vi "ExampleAll.vi"() -> ()   [LabVIEW 2009]
uses:
  Shamrock.llb/shamrock_flipperPort_typedef.ctl
  Shamrock.llb/shamrock_lipperMirror_typedef.ctl
  C/Program Files (x86)/National Instruments/LabVIEW 2018/user.lib/Shamrock.llb/shamrock_autoSlit_typedef.ctl
panel:
  in  "Device":i32 min=0 max=1
  in  "Tab Control":T1(tab)
  in  "Grating Offset":i32
  out "SetGratingOffset":string
  in  "Detector Offset":i32
  out "SetDetectorOffset":string
  out "WavelengthReset":string
  out "SetGrating":string
  in  "Grating":i32
  in  "Turret":i32
  out "SetTurret":string
  in  "SetGratingOffset":bool
  in  "SetDetectorOffset":bool
  in  "WavelengthReset":bool
  in  "SetGrating":bool
  in  "SetTurret":bool
  out "blaze":string
  out "Grating Offset":i32
  out "Detector Offset":i32
  out "offset":i32
  out "home":i32
  out "lines/mm":dbl format="%.2f"
  out "Grating":i32
  out "No Gratings":i32
  out "Turret":i32
  out "Is Grating ?":string
  out "GetGratingOffset":string
  out "GetDetectorOffset":string
  out "GetGratingInfo":string
  out "GetGrating":string
  out "GetNumberGratings":string
  out "GetTurret":string
  out "GratingIsPresent":string
  out "GetCalibration":string
  out "SetNumberPixels":string
  out "SetPixelWidth":string
  out "Max Dispersion":sgl
  out "Min Dispersion":sgl
  in  "Number Pixels":u32 caption="Numeric"
  in  "Pixel Width":sgl caption="Numeric" format="%_3g"
  out "GotoZeroOrder":string
  out "SetWavelength":string
  in  "Wavelength":dbl format="%.2f"
  in  "GoToZeroOrder":bool
  out "Max Wavelength":dbl format="%.2f"
  out "Min Wavelength":dbl format="%.2f"
  out "Is Wavelength ?":string
  out "WavelengthIsPresent":string
  out "GetWavelengthLimits":string
  out "At Zero Order ?":string
  out "AtZeroOrder":string
  out "Wavelength":dbl format="%.2f"
  in  "SetWavelength 2":bool
  out "GetWavelength":string
  out "SetSlitZeroPosition":string
  out "GetSlitZeroPosition":string
  in  "SlitZeroPositionSet":bool caption="SetSlitZeroPosition"
  in  "SlitZeroPositionGet":bool
  in  "SlitZeroPosition":i32
  in  "Reset Slit":bool
  out "ResetSlit":string
  out "Getslit":string
  in  "Slit Width":dbl format="%.2f"
  in  "SetSlit":bool
  out "Slit width(mm)":dbl format="%.2f"
  out "GetSlit":string
  out "SlitIsPresent retun code":string
  in  "Slit":T2
  out "Is Slit Present?":bool
  in  "Mode":i32
  in  "SetShutter":bool
  out "Is Mode Possible ?":string
  out "Shutter":i32
  out "Is Shutter ?":string
  out "SetShutter":string
  out "IsModePossible":string
  out "GetShutter":string
  out "ShutterIsPresent":string
  in  "Flipper Port":T3
  out "High":dbl format="%.2f"
  in  "FlipperReset":bool
  out "FlipperReset":string
  in  "SetPort":bool
  out "Low":dbl format="%.2f"
  out "Port":T3
  out "Is Flipper ?":string
  out "SetPort":string
  out "GetCCDLimits":string
  out "GetPort":string
  out "FlipperIsPresent":string
  out "GetFlipperMirror":string
  in  "FlipperSelect":bool
  in  "Flipper Mirror":T4
  in  "Filter info":string caption="String"
  out "Filter Info":string
  in  "SetFilterInfo":bool
  out "SetFilterInfo":string
  in  "Filter":i32
  in  "SetFilter":bool
  out "Filter":i32
  out "Is Filter ?":string
  out "SetFilter":string
  out "GetFilterInfo":string
  out "GetFilter":string
  out "FilterIsPresent":string
  in  "Reset Focus Mirror":bool
  out "Is Focus Mirror Present?":bool
  out "Focus Mirror Max Steps":i32
  in  "Focus Mirror -":bool
  in  "Focus":i32
  in  "Focus Mirror +":bool
  out "Focus Mirror Position":i32
  out "GetFocusMirrorMaxSteps":string
  out "GetFocusMirror":string
  out "FocusMirrorIsPresent":string
  in  "Line":i32
  out "Line 2":i32
  in  "State":i32
  in  "Set Accessory":bool
  out "Line 1":i32
  out "Is Accessory ?":string
  out "SetAccessory":string
  out "GetAccessory":string
  out "AccessoryIsPresent":string
  in  "Set Params":bool
  out "Set Optical Parameters":string
  in  "Focal tilt":dbl format="%.2f"
  in  "Angular deviation":dbl format="%.2f"
  in  "Focal length":dbl format="%.4f"
  out "Initializing":bool
  in  "STOP if TRUE":bool
  out "Focal tilt":dbl format="%.2f"
  out "Angular deviation":dbl format="%.2f"
  out "Focal length":dbl format="%.4f"
  out "Serial Number":string
  out "No of devices":i32
  out "GetOpticalParameters":string
  out "GetSerialNumber":string
  out "GetNumberDevices":string
  out "Close":string
  out "Initialize":string
  # "INITIALIZATION"
  # "SDK RETURN VALUES"
  # "SHAMROCK PARAMETERS"
  # "ACTIONS"
  # "SDK RETURN VALUES"
  # "SHAMROCK PARAMETERS"
  # "ACTIONS"
  # "SDK RETURN VALUES"
  # "SHAMROCK PARAMETERS"
  # "ACTIONS"
  # "nm"
  # "Dispersion range"
  # "SDK RETURN VALUES"
  # "SHAMROCK PARAMETERS"
  # "ACTIONS"
  # "mm"
  # "SetZero position"
  # "SDK RETURN VALUES"
  # "SHAMROCK PARAMETERS"
  # "ACTIONS"
  # "( 0:Closed / 1:Open )"
  # "SDK RETURN VALUES"
  # "SHAMROCK PARAMETERS"
  # "ACTIONS"
  # "SDK RETURN VALUES"
  # "SHAMROCK PARAMETERS"
  # "ACTIONS"
  # "SDK RETURN VALUES"
  # "SHAMROCK PARAMETERS"
  # "ACTIONS"
  # "SDK RETURN VALUES"
  # "SHAMROCK PARAMETERS"
  # "ACTIONS"
  # "line"
  # "to state"
  # "SDK RETURN VALUES"
  # "SHAMROCK PARAMETERS"
  # "ACTIONS"
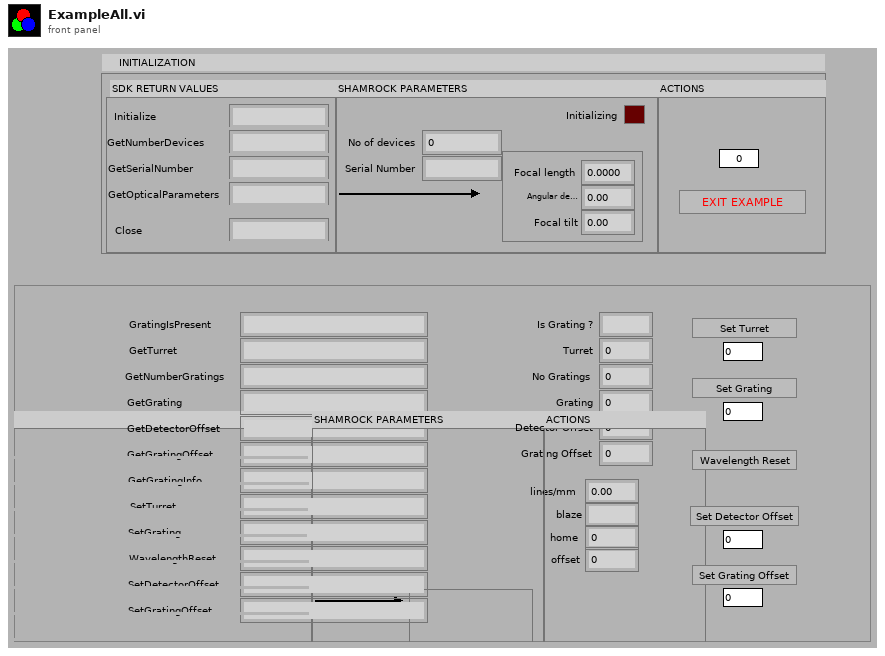
[diagram p1: front panel]
types:
  T1 = enum32{"GRATINGS", "WAVELENGTH", "INPUT & OUTPUT SLIT", "SHUTTER", "FLIPPER", "FILTER", "FOCUS", "ACCESSORY", "OPTICALPARAMS"}
  T2 = typedef "shamrock_autoSlit_typedef.ctl" = enum32{"Reserved (0)", "INPUT SIDE", "INPUT DIRECT", "OUTPUT SIDE", "OUTPUT DIRECT"}
  T3 = typedef "shamrock_flipperPort_typedef.ctl" = enum32{"DIRECT PORT", "SIDE PORT"}
  T4 = typedef "shamrock_lipperMirror_typedef.ctl" = enum32{"Reserved (0)", "INPUT MIRROR", "OUTPUT MIRROR"}
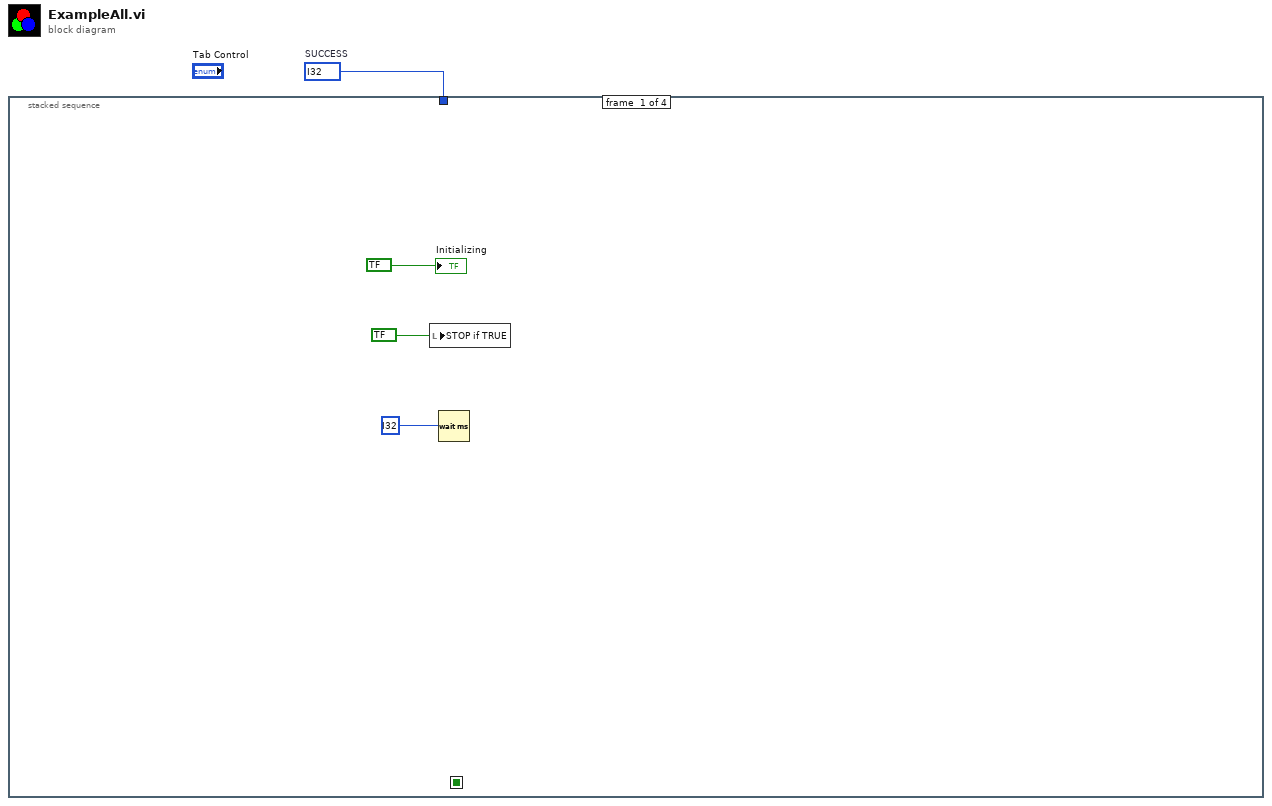
[diagram p0: block diagram]
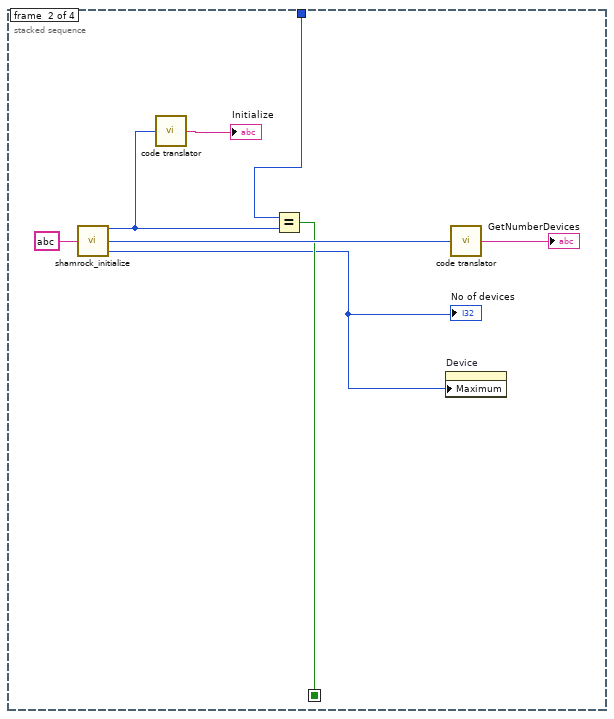
[diagram p2: hidden frame]
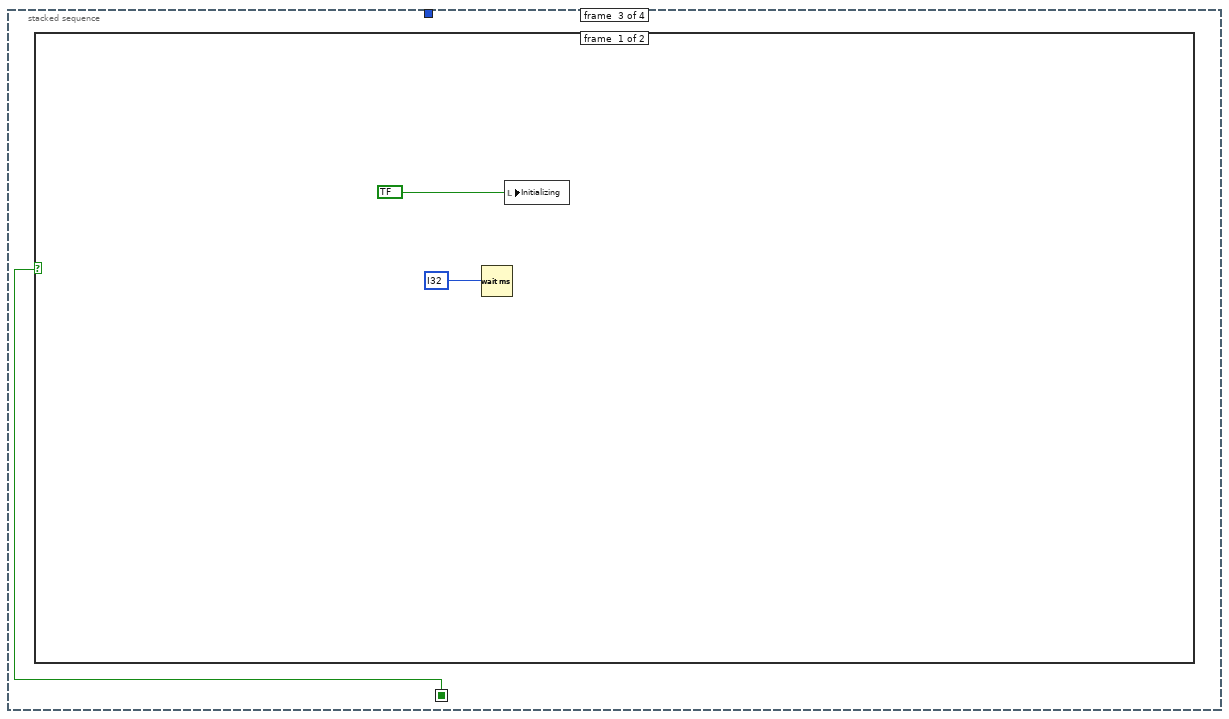
[diagram p3: hidden frame]
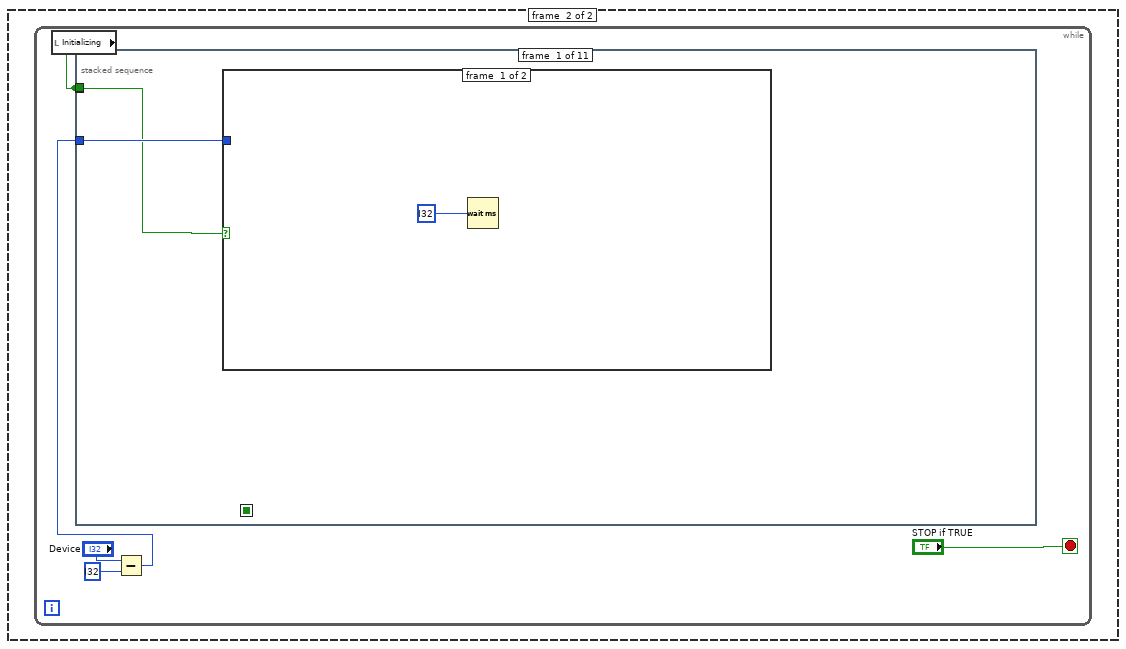
[diagram p4: hidden frame]
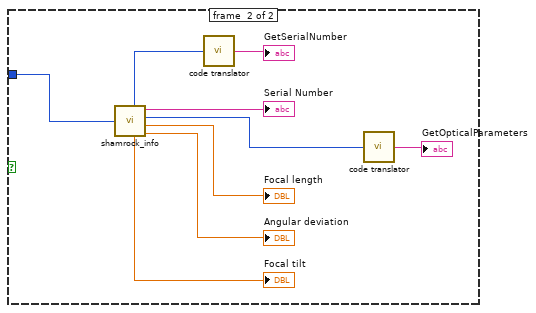
[diagram p5: hidden frame]
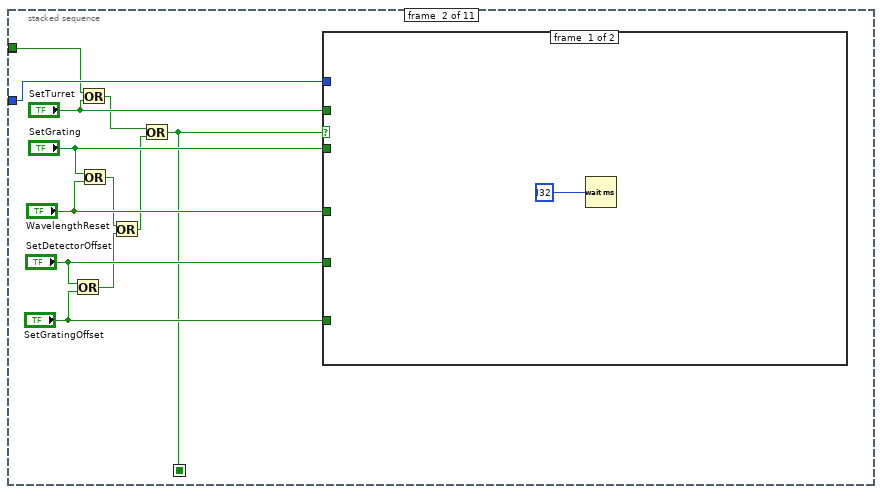
[diagram p6: hidden frame]
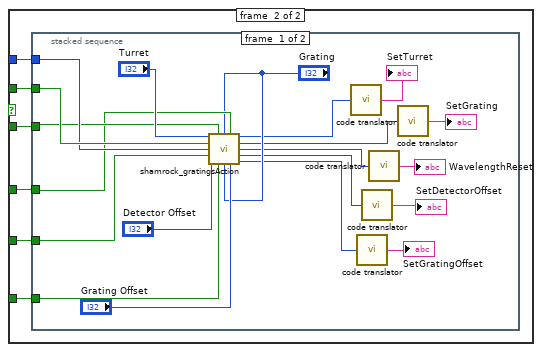
[diagram p7: hidden frame]
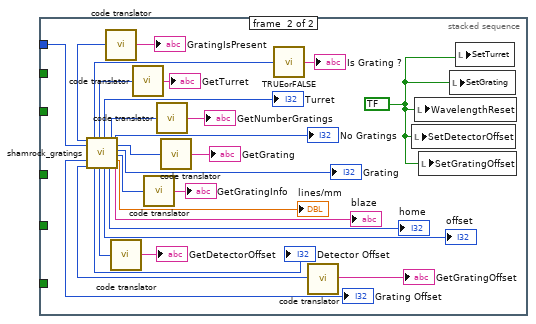
[diagram p8: hidden frame]
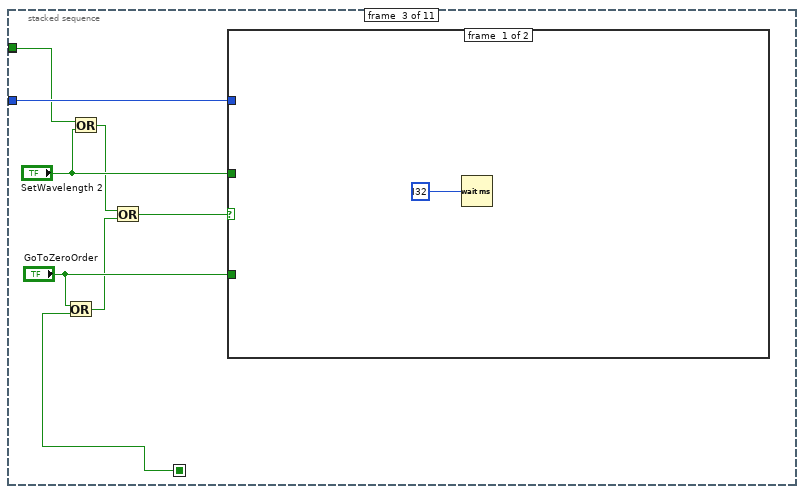
[diagram p9: hidden frame]
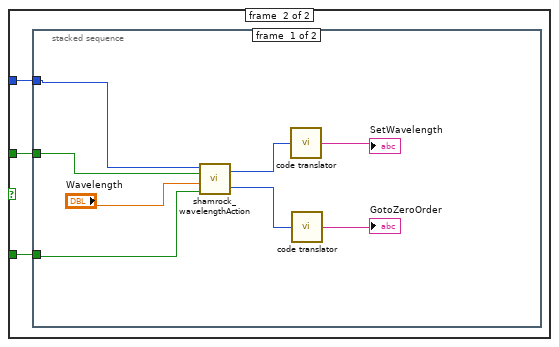
[diagram p10: hidden frame]
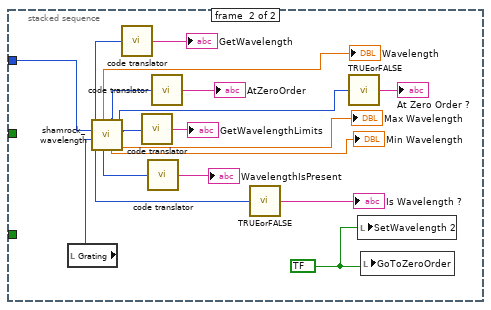
[diagram p11: hidden frame]
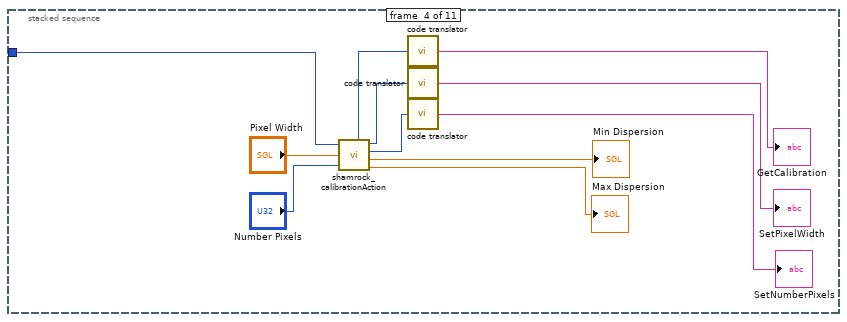
[diagram p12: hidden frame]
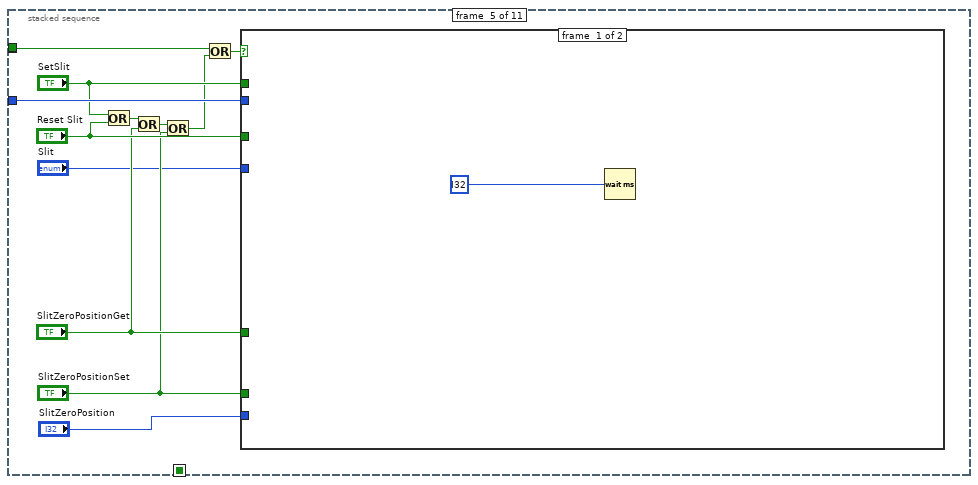
[diagram p13: hidden frame]
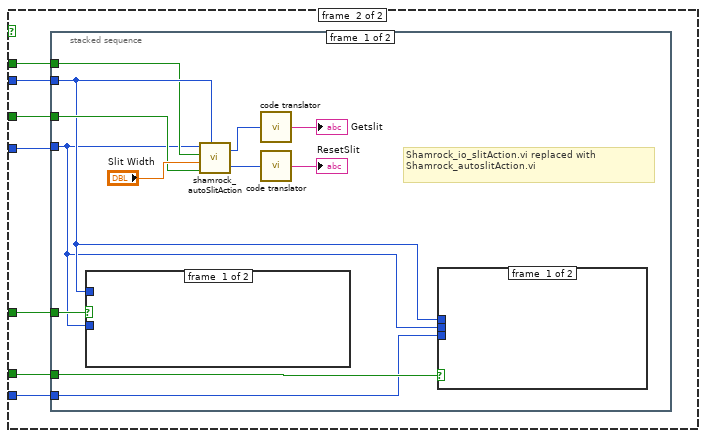
[diagram p14: hidden frame]
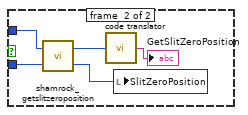
[diagram p15: hidden frame]
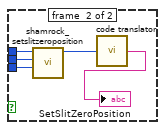
[diagram p16: hidden frame]
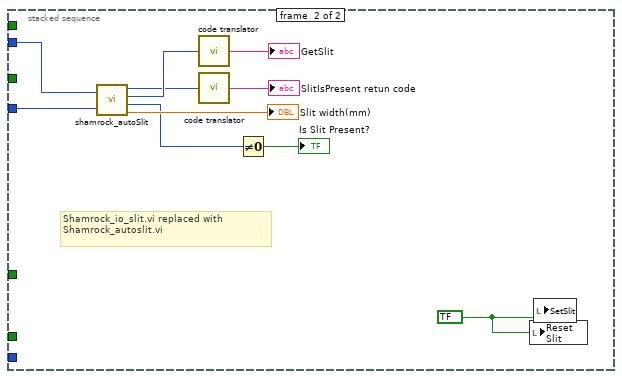
[diagram p17: hidden frame]
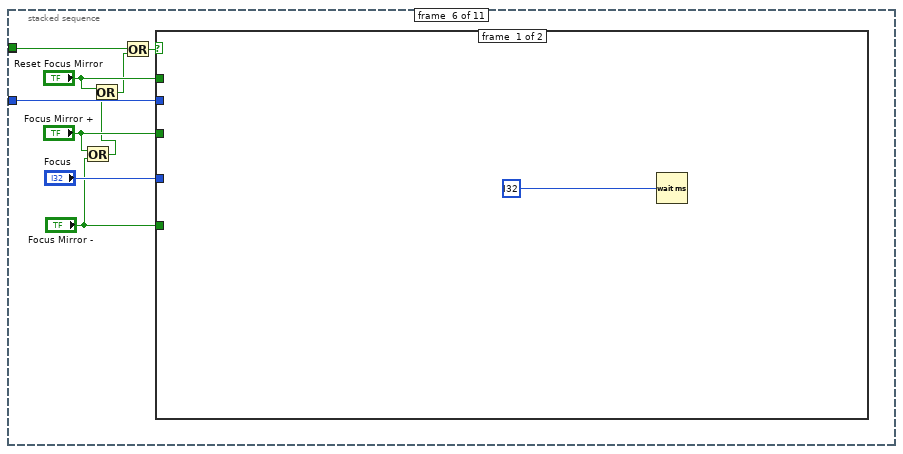
[diagram p18: hidden frame]
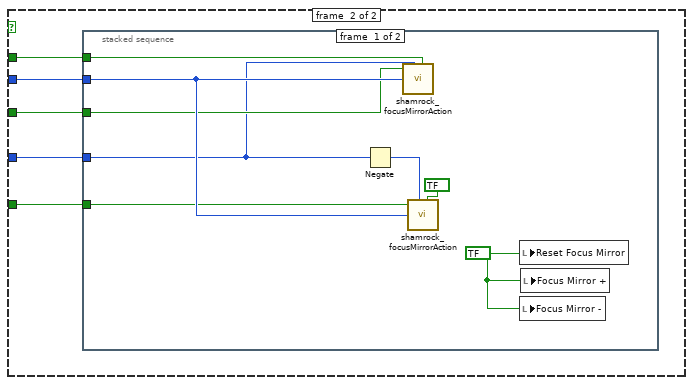
[diagram p19: hidden frame]
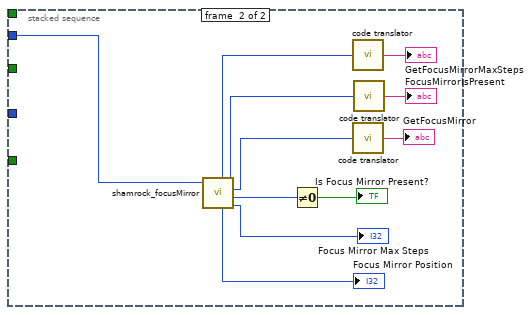
[diagram p20: hidden frame]
diagram:
  w1 = i32 ?  # SUCCESS
  n1 = stacked-sequence {
    seq-local: [_ w6 _ _] -> [_ _ w13 _]
    tunnel: w1 -> [_ w12 _ _]
    frame #0 {
      n2 = local write "STOP if TRUE"(bool ?) -> ()
      n3 = Wait (ms)(milliseconds to wait=i32 ?) -> ()  [unwired: 1 out]
      "Initializing" <- bool ?
    }
    frame #1 {
      n4 = call "shamrock_initialize.vi"("Initialization path"=string ?) -> ("Initialize"=w9:u32, "GetNumberDevices"=w8:u32, "No of devices"=w5:i32)
      "No of devices" <- w5
      n5 = call "code translator.vi"("Error code"=w9) -> ("Error description"=→"Initialize":string)
      n6 = Equal?(x=w12, y=w9) -> (x = y?=w6:bool)
      n7 = property on="Device" class="DigNum (strict)"("Maximum"=w5) -> ()  [unwired: 2 in, 2 out]
      n8 = call "code translator.vi"("Error code"=w8) -> ("Error description"=→"GetNumberDevices":string)
    }
    frame #2 {
      n9 = case shown="True" w13 {
        frame #0 {
          n10 = Wait (ms)(milliseconds to wait=i32 ?) -> ()  [unwired: 1 out]
          n11 = local write "Initializing"(bool ?) -> ()
        }
        frame #1 {
          n12 = while {
            stop <- "STOP if TRUE" stop-if-true
            n13 = local read "Initializing"() -> (w16:bool)
            n14 = Subtract(x="Device", y=i32 ?) -> (x-y=w19:i32)
            n15 = stacked-sequence {
              seq-local: [_ w33 _ _ _ _ _ _ _ _ _] -> [_ _ w105 _ _ _ _ _ _ _ _]
              tunnel: w19 -> [w22 w44 w106 w138 w159 w208 w237 w267 w302 w331 w355]
              tunnel: w16 -> [w21 w36 w102 _ w155 w201 w234 _ w297 w328 _]
              tunnel: w16 -> [_ _ _ _ _ _ _ w263 _ _ _]
              frame #0 {
                n16 = case shown="True" w21 {
                  tunnel: w22 -> [_ w24]
                  frame #0 {
                    n17 = Wait (ms)(milliseconds to wait=i32 ?) -> ()  [unwired: 1 out]
                  }
                  frame #1 {
                    n18 = call "shamrock_info.vi"("Device No"=w24) -> ("GetSerialNumber"=w28:u32, "Focal tilt"=→"Focal tilt":sgl, "Serial Number"=→"Serial Number":string, "GetOpticalParameters"=w26:u32, "Focal length"=→"Focal length":sgl, "Angular deviation"=→"Angular deviation":sgl)
                    n19 = call "code translator.vi"("Error code"=w28) -> ("Error description"=→"GetSerialNumber":string)
                    n20 = call "code translator.vi"("Error code"=w26) -> ("Error description"=→"GetOpticalParameters":string)
                  }
                }
              }
              frame #1 {
                n21 = Or(x="SetDetectorOffset", y="SetGratingOffset") -> (x .or. y?=w38:bool)
                n22 = Or(x=w36, y="SetTurret") -> (x .or. y?=w35:bool)
                n23 = Or(x="SetGrating", y="WavelengthReset") -> (x .or. y?=w39:bool)
                n24 = Or(x=w39, y=w38) -> (x .or. y?=w34:bool)
                n25 = Or(x=w35, y=w34) -> (x .or. y?=w33:bool)
                n26 = case shown="True" w33 {
                  tunnel: w44 -> [_ w51]
                  tunnel: "SetDetectorOffset" -> [_ w50]
                  tunnel: "SetGratingOffset" -> [_ w49]
                  tunnel: "SetGrating" -> [_ w48]
                  tunnel: "WavelengthReset" -> [_ w47]
                  tunnel: "SetTurret" -> [_ w46]
                  frame #0 {
                    n27 = Wait (ms)(milliseconds to wait=i32 ?) -> ()  [unwired: 1 out]
                  }
                  frame #1 {
                    n28 = stacked-sequence {
                      tunnel: w46 -> [w70 _]
                      tunnel: w51 -> [w69 w89]
                      tunnel: w48 -> [w64 _]
                      tunnel: w47 -> [w63 _]
                      tunnel: w50 -> [w68 _]
                      tunnel: w49 -> [w66 _]
                      frame #0 {
                        n29 = call "shamrock_gratingsAction.vi"("WavelengthReset"=w63, "Grating Offset"="Grating Offset", 7:"Grating"="Grating", 8:"Grating"="Grating", "SetGrating"=w64, "SetGratingOffset"=w66, "Turret"="Turret", "SetTurret"=w70, "Device No"=w69, "SetDetectorOffset"=w68, "Detector Offset"="Detector Offset") -> ("SetTurret"=w61:u32, "SetGrating"=w59:u32, "WavelengthReset"=w56:u32, "SetDetectorOffset"=w54:u32, "SetGratingOffset"=w53:u32)
                        n30 = call "code translator.vi"("Error code"=w61) -> ("Error description"=→"SetTurret":string)
                        n31 = call "code translator.vi"("Error code"=w53) -> ("Error description"=→"SetGratingOffset":string)
                        n32 = call "code translator.vi"("Error code"=w54) -> ("Error description"=→"SetDetectorOffset":string)
                        n33 = call "code translator.vi"("Error code"=w56) -> ("Error description"=→"WavelengthReset":string)
                        n34 = call "code translator.vi"("Error code"=w59) -> ("Error description"=→"SetGrating":string)
                      }
                      frame #1 {
                        w98 = bool ?
                        n35 = call "shamrock_gratings.vi"("Device No"=w89) -> ("No Gratings"=→"No Gratings":i32, "GetNumberGratings"=w83:u32, "Turret"=→"Turret":i32, "GetTurret"=w85:u32, "0:FALSE / 1:TRUE"=w73:i32, "GratingIsPresent"=w87:u32, "GetGrating"=w81:u32, "Grating"=→"Grating":i32, "GetGratingInfo"=w79:u32, "lines/mm"=→"lines/mm":dbl, "Grating Offset"=→"Grating Offset":i32, "blaze"=→"blaze":string, "home"=→"home":i32, "offset"=→"offset":i32, "GetDetectorOffset"=w77:u32, "Detector Offset"=→"Detector Offset":i32, "GetGratingOffset"=w75:u32)  [unwired: 1 in, 1 out]
                        n36 = call "code translator.vi"("Error code"=w87) -> ("Error description"=→"GratingIsPresent":string)
                        n37 = call "code translator.vi"("Error code"=w77) -> ("Error description"=→"GetDetectorOffset":string)
                        n38 = call "code translator.vi"("Error code"=w85) -> ("Error description"=→"GetTurret":string)
                        n39 = call "code translator.vi"("Error code"=w79) -> ("Error description"=→"GetGratingInfo":string)
                        n40 = call "code translator.vi"("Error code"=w83) -> ("Error description"=→"GetNumberGratings":string)
                        n41 = call "code translator.vi"("Error code"=w81) -> ("Error description"=→"GetGrating":string)
                        n42 = call "TRUEorFALSE.vi"("bool number"=w73) -> ("String"=→"Is Grating ?":string)
                        n43 = call "code translator.vi"("Error code"=w75) -> ("Error description"=→"GetGratingOffset":string)
                        n44 = local write "SetDetectorOffset"(w98) -> ()
                        n45 = local write "WavelengthReset"(w98) -> ()
                        n46 = local write "SetGratingOffset"(w98) -> ()
                        n47 = local write "SetGrating"(w98) -> ()
                        n48 = local write "SetTurret"(w98) -> ()
                      }
                    }
                  }
                }
              }
              frame #2 {
                n49 = Or(x="GoToZeroOrder", y=w105) -> (x .or. y?=w100:bool)
                n50 = Or(x=w102, y="SetWavelength 2") -> (x .or. y?=w101:bool)
                n51 = Or(x=w101, y=w100) -> (x .or. y?=w99:bool)
                n52 = case shown="True" w99 {
                  tunnel: "SetWavelength 2" -> [_ w110]
                  tunnel: "GoToZeroOrder" -> [_ w109]
                  tunnel: w106 -> [_ w108]
                  frame #0 {
                    n53 = Wait (ms)(milliseconds to wait=i32 ?) -> ()  [unwired: 1 out]
                  }
                  frame #1 {
                    n54 = stacked-sequence {
                      tunnel: w110 -> [w116 _]
                      tunnel: w109 -> [w117 _]
                      tunnel: w108 -> [w115 w131]
                      frame #0 {
                        n55 = call "shamrock_wavelengthAction.vi"("GoToZeroOrder"=w117, "Wavelength"="Wavelength", "SetWavelength"=w116, "Device No"=w115) -> ("GotoZeroOrder"=w112:u32, "SetWavelength"=w114:u32)
                        n56 = call "code translator.vi"("Error code"=w114) -> ("Error description"=→"SetWavelength":string)
                        n57 = call "code translator.vi"("Error code"=w112) -> ("Error description"=→"GotoZeroOrder":string)
                      }
                      frame #1 {
                        w136 = bool ?
                        n58 = local read "Grating"() -> (w132:i32)
                        n59 = call "shamrock_wavelength.vi"("Grating No"=w132, "Device No"=w131) -> (0:"0:FALSE / 1:TRUE"=w120:i32, "WavelengthIsPresent"=w124:u32, "Min wl"=→"Min Wavelength":dbl, "Max wl"=→"Max Wavelength":dbl, "GetWavelengthLimits"=w126:u32, "GetWavelength"=w130:u32, "Wavelength"=→"Wavelength":dbl, "AtZeroOrder"=w128:u32, 10:"0:FALSE / 1:TRUE"=w122:i32)
                        n60 = call "code translator.vi"("Error code"=w130) -> ("Error description"=→"GetWavelength":string)
                        n61 = call "code translator.vi"("Error code"=w126) -> ("Error description"=→"GetWavelengthLimits":string)
                        n62 = call "code translator.vi"("Error code"=w124) -> ("Error description"=→"WavelengthIsPresent":string)
                        n63 = call "code translator.vi"("Error code"=w128) -> ("Error description"=→"AtZeroOrder":string)
                        n64 = call "TRUEorFALSE.vi"("bool number"=w120) -> ("String"=→"Is Wavelength ?":string)
                        n65 = call "TRUEorFALSE.vi"("bool number"=w122) -> ("String"=→"At Zero Order ?":string)
                        n66 = local write "SetWavelength 2"(w136) -> ()
                        n67 = local write "GoToZeroOrder"(w136) -> ()
                      }
                    }
                  }
                }
              }
              frame #3 {
                n68 = call "shamrock_calibrationAction.vi"("Set Number Pixels"="Number Pixels", "Set Pixel Width"="Pixel Width", "Device No"=w138) -> ("Wavelength Last Pixel"=→"Max Dispersion":sgl, "Wavelength First Pixel"=→"Min Dispersion":sgl, "Set Number Pixels"=w143:u32, "GetCalibration"=w147:u32, "Set Pixel Width"=w145:u32)  [unwired: 1 out]
                n69 = call "code translator.vi"("Error code"=w147) -> ("Error description"=→"GetCalibration":string)
                n70 = call "code translator.vi"("Error code"=w145) -> ("Error description"=→"SetPixelWidth":string)
                n71 = call "code translator.vi"("Error code"=w143) -> ("Error description"=→"SetNumberPixels":string)
              }
              frame #4 {
                n72 = Or(x="SetSlit", y="Reset Slit") -> (x .or. y?=w148:bool)
                n73 = Or(x=w148, y="SlitZeroPositionGet") -> (x .or. y?=w150:bool)
                n74 = Or(x=w150, y="SlitZeroPositionSet") -> (x .or. y?=w151:bool)
                n75 = Or(x=w155, y=w151) -> (x .or. y?=w156:bool)
                n76 = case shown="True" w156 {
                  tunnel: w159 -> [_ w167]
                  tunnel: "SetSlit" -> [_ w166]
                  tunnel: "Reset Slit" -> [_ w165]
                  tunnel: "SlitZeroPositionGet" -> [_ w164]
                  tunnel: "SlitZeroPositionSet" -> [_ w163]
                  tunnel: "SlitZeroPosition" -> [_ w162]
                  tunnel: "Slit" -> [_ w161]
                  frame #0 {
                    n77 = Wait (ms)(milliseconds to wait=i32 ?) -> ()  [unwired: 1 out]
                  }
                  frame #1 {
                    n78 = stacked-sequence {
                      tunnel: w166 -> [w169 _]
                      tunnel: w167 -> [w172 w196]
                      tunnel: w165 -> [w173 _]
                      tunnel: w164 -> [w177 _]
                      tunnel: w163 -> [w176 _]
                      tunnel: w162 -> [w175 _]
                      tunnel: w161 -> [w168 w195]
                      frame #0 {
                        # "Shamrock_io_slitAction.vi replaced with \nShamrock_autoslitAction.vi"
                        n79 = case shown="True" w177 {
                          tunnel: w172 -> [_ w183]
                          tunnel: w168 -> [_ w182]
                          frame #0 {
                          }
                          frame #1 {
                            n80 = call "shamrock_getslitzeroposition.vi"("Slit Index"=w182, "Device No"=w183) -> ("Offset"=w180:i32, "GetSlitZeroPosition"=w181:u32)
                            n81 = call "code translator.vi"("Error code"=w181) -> ("Error description"=→"GetSlitZeroPosition":string)
                            n82 = local write "SlitZeroPosition"(w180) -> ()
                          }
                        }
                        n83 = call "shamrock_autoSlitAction.vi"("Slit"=w168, "SetSlit"=w169, "Slit Width"="Slit Width", "Reset Slit"=w173, "Device No"=w172) -> ("RC_ResetSlit"=w170:u32, "RC_SetSlit"=w171:u32)
                        n84 = call "code translator.vi"("Error code"=w170) -> ("Error description"=→"Getslit":string)
                        n85 = call "code translator.vi"("Error code"=w171) -> ("Error description"=→"ResetSlit":string)
                        n86 = case shown="True" w176 {
                          tunnel: w172 -> [_ w188]
                          tunnel: w168 -> [_ w187]
                          tunnel: w175 -> [_ w186]
                          frame #0 {
                          }
                          frame #1 {
                            n87 = call "shamrock_setslitzeroposition.vi"("Offset"=w186, "Slit Index"=w187, "Device No"=w188) -> ("SetSlitZeroPosition"=w185:u32)  [unwired: 7 in]
                            n88 = call "code translator.vi"("Error code"=w185) -> ("Error description"=→"SetSlitZeroPosition":string)
                          }
                        }
                      }
                      frame #1 {
                        w199 = bool ?
                        # "Shamrock_io_slit.vi replaced with \nShamrock_autoslit.vi"
                        n89 = call "shamrock_autoSlit.vi"("Device No"=w196, "Slit"=w195) -> ("RC_SlitIsPresent"=w192:u32, "RC_GetSlit"=w194:u32, "IsPresent"=w191:i32, "Slit width (mm)"=→"Slit width(mm)":dbl)
                        n90 = call "code translator.vi"("Error code"=w194) -> ("Error description"=→"GetSlit":string)
                        n91 = call "code translator.vi"("Error code"=w192) -> ("Error description"=→"SlitIsPresent retun code":string)
                        n92 = Not Equal To 0?(x=w191) -> (x != 0?=→"Is Slit Present?":bool)
                        n93 = local write "Reset Slit"(w199) -> ()
                        n94 = local write "SetSlit"(w199) -> ()
                      }
                    }
                  }
                }
              }
              frame #5 {
                n95 = Or(x="Focus Mirror +", y="Focus Mirror -") -> (x .or. y?=w203:bool)
                n96 = Or(x="Reset Focus Mirror", y=w203) -> (x .or. y?=w200:bool)
                n97 = Or(x=w201, y=w200) -> (x .or. y?=w202:bool)
                n98 = case shown="True" w202 {
                  tunnel: w208 -> [_ w214]
                  tunnel: "Focus Mirror +" -> [_ w213]
                  tunnel: "Focus Mirror -" -> [_ w212]
                  tunnel: "Focus" -> [_ w211]
                  tunnel: "Reset Focus Mirror" -> [_ w210]
                  frame #0 {
                    n99 = Wait (ms)(milliseconds to wait=i32 ?) -> ()  [unwired: 1 out]
                  }
                  frame #1 {
                    n100 = stacked-sequence {
                      tunnel: w214 -> [w219 w223]
                      tunnel: w213 -> [w218 _]
                      tunnel: w212 -> [w217 _]
                      tunnel: w211 -> [w216 _]
                      tunnel: w210 -> [w215 _]
                      frame #0 {
                        w220 = bool ?
                        n101 = Negate(x=w216) -> (-x=w222:i32)
                        n102 = call "shamrock_focusMirrorAction.vi"("Set Focus Mirror"=w218, "Focus"=w216, "Device No"=w219, "Reset Focus Mirror"=w215) -> ()  [unwired: 5 in, 2 out]
                        n103 = call "shamrock_focusMirrorAction.vi"("Set Focus Mirror"=w217, "Focus"=w222, "Device No"=w219, "Reset Focus Mirror"=bool ?) -> ()  [unwired: 5 in, 2 out]
                        n104 = local write "Reset Focus Mirror"(w220) -> ()
                        n105 = local write "Focus Mirror -"(w220) -> ()
                        n106 = local write "Focus Mirror +"(w220) -> ()
                      }
                      frame #1 {
                        n107 = call "shamrock_focusMirror.vi"("Device No"=w223) -> ("Max Step Position"=→"Focus Mirror Max Steps":i32, "Current Step Position"=→"Focus Mirror Position":i32, "IsPresent"=w233:i32, "RC_GetFocusMirror"=w228:u32, "RC_GetFocusMirrorMax"=w227:u32, "RC_FocusMirrorPresent"=w226:u32)  [unwired: 2 in]
                        n108 = Not Equal To 0?(x=w233) -> (x != 0?=→"Is Focus Mirror Present?":bool)
                        n109 = call "code translator.vi"("Error code"=w227) -> ("Error description"=→"GetFocusMirrorMaxSteps":string)
                        n110 = call "code translator.vi"("Error code"=w228) -> ("Error description"=→"GetFocusMirror":string)
                        n111 = call "code translator.vi"("Error code"=w226) -> ("Error description"=→"FocusMirrorIsPresent":string)
                      }
                    }
                  }
                }
              }
              frame #6 {
                n112 = Or(x=w234, y="SetShutter") -> (x .or. y?=w235:bool)
                n113 = case shown="True" w235 {
                  tunnel: w237 -> [_ w240]
                  tunnel: "SetShutter" -> [_ w239]
                  frame #0 {
                    n114 = Wait (ms)(milliseconds to wait=i32 ?) -> ()  [unwired: 1 out]
                  }
                  frame #1 {
                    n115 = stacked-sequence {
                      seq-local: ["Mode" _] -> [_ w256]
                      tunnel: w240 -> [w243 w257]
                      tunnel: w239 -> [w244 _]
                      frame #0 {
                        n116 = call "shamrock_shutterAction.vi"("Mode"="Mode", "SetShutter"=w244, "Device No"=w243) -> ("SetShutter"=w242:u32)
                        n117 = call "code translator.vi"("Error code"=w242) -> ("Error description"=→"SetShutter":string)
                      }
                      frame #1 {
                        n118 = call "shamrock_shutter.vi"("Device No"=w257, "Mode"=w256) -> ("ShutterIsPresent"=w255:u32, 3:"0:FALSE / 1:TRUE"=w247:i32, 4:"0:FALSE / 1:TRUE"=w248:i32, "GetShutter"=w253:u32, "Shutter"=→"Shutter":i32, "IsModePossible"=w251:u32)
                        n119 = call "code translator.vi"("Error code"=w255) -> ("Error description"=→"ShutterIsPresent":string)
                        n120 = call "code translator.vi"("Error code"=w251) -> ("Error description"=→"IsModePossible":string)
                        n121 = call "code translator.vi"("Error code"=w253) -> ("Error description"=→"GetShutter":string)
                        n122 = call "TRUEorFALSE.vi"("bool number"=w247) -> ("String"=→"Is Mode Possible ?":string)
                        n123 = call "TRUEorFALSE.vi"("bool number"=w248) -> ("String"=→"Is Shutter ?":string)
                        n124 = local write "SetShutter"(bool ?) -> ()
                      }
                    }
                  }
                }
              }
              frame #7 {
                n125 = Or(x="SetPort", y="FlipperReset") -> (x .or. y?=w264:bool)
                n126 = Or(x=w263, y=w264) -> (x .or. y?=w262:bool)
                n127 = Or(x=w262, y="FlipperSelect") -> (x .or. y?=w260:bool)
                n128 = case shown="True" w260 {
                  tunnel: "SetPort" -> [_ w272]
                  tunnel: "FlipperReset" -> [_ w271]
                  tunnel: w267 -> [_ w270]
                  frame #0 {
                    n129 = Wait (ms)(milliseconds to wait=i32 ?) -> ()  [unwired: 1 out]
                  }
                  frame #1 {
                    n130 = stacked-sequence {
                      tunnel: w272 -> [w275 _]
                      tunnel: w271 -> [w274 _]
                      tunnel: w270 -> [w277 w291]
                      tunnel: "Flipper Mirror" -> [w276 w290]
                      frame #0 {
                        n131 = call "shamrock_flipperMirrorAction.vi"(0:w276, "SetPort"=w275, 2:"Flipper Port", "FlipperReset"=w274, "Device No"=w277) -> ("RC_SetPort"=w281:u32, "RC_FlipperReset"=w280:u32)
                        n132 = call "code translator.vi"("Error code"=w281) -> ("Error description"=→"SetPort":string)
                        n133 = call "code translator.vi"("Error code"=w280) -> ("Error description"=→"FlipperReset":string)
                      }
                      frame #1 {
                        w296 = bool ?
                        n134 = call "shamrock_flipperMirror.vi"("Flipper"=w290, "Device No"=w291) -> ("High"=→"High":dbl, "RC_GetCCDLimits"=w287:u32, "Low"=→"Low":dbl, "Flipper Port"=w282:T3, "RC_GetFlipperMirror"=w284:u32, "IsPresent"=w283:i32, "RC_FlipperIsPresent"=w286:u32)
                        "Port" <- w282
                        n135 = call "code translator.vi"("Error code"=w284) -> ("Error description"=→"GetFlipperMirror":string)
                        n136 = call "code translator.vi"("Error code"=w287) -> ("Error description"=→"GetCCDLimits":string)
                        n137 = call "code translator.vi"("Error code"=w286) -> ("Error description"=→"FlipperIsPresent":string)
                        n138 = call "code translator.vi"("Error code"=w282) -> ("Error description"=→"GetPort":string)
                        n139 = local write "SetPort"(w296) -> ()
                        n140 = local write "FlipperReset"(w296) -> ()
                        n141 = call "TRUEorFALSE.vi"("bool number"=w283) -> ("String"=→"Is Flipper ?":string)
                      }
                    }
                  }
                }
              }
              frame #8 {
                n142 = Or(x="SetFilter", y="SetFilterInfo") -> (x .or. y?=w299:bool)
                n143 = Or(x=w297, y=w299) -> (x .or. y?=w298:bool)
                n144 = case shown="True" w298 {
                  tunnel: w302 -> [_ w306]
                  tunnel: "SetFilter" -> [_ w305]
                  tunnel: "SetFilterInfo" -> [_ w304]
                  frame #0 {
                    n145 = Wait (ms)(milliseconds to wait=i32 ?) -> ()  [unwired: 1 out]
                  }
                  frame #1 {
                    n146 = stacked-sequence {
                      tunnel: w306 -> [w312 w324]
                      tunnel: w305 -> [w315 _]
                      tunnel: w304 -> [w314 _]
                      frame #0 {
                        n147 = call "shamrock_filterAction.vi"("Filter info"="Filter info", "Device No"=w312, 4:"Filter"="Filter", "SetFilterInfo"=w314, 6:"Filter"="Filter", "SetFilter"=w315) -> ("SetFilterInfo"=w307:u32, "SetFilter"=w310:u32)
                        n148 = call "code translator.vi"("Error code"=w310) -> ("Error description"=→"SetFilter":string)
                        n149 = call "code translator.vi"("Error code"=w307) -> ("Error description"=→"SetFilterInfo":string)
                      }
                      frame #1 {
                        w327 = bool ?
                        n150 = call "shamrock_filter.vi"("Device No"=w324) -> ("FilterIsPresent"=w323:u32, "Filter Info"=→"Filter Info":string, "0:FALSE / 1:TRUE"=w316:i32, "GetFilter"=w321:u32, "Filter"=→"Filter":i32, "GetFilterInfo"=w319:u32)
                        n151 = call "code translator.vi"("Error code"=w323) -> ("Error description"=→"FilterIsPresent":string)
                        n152 = call "code translator.vi"("Error code"=w319) -> ("Error description"=→"GetFilterInfo":string)
                        n153 = call "code translator.vi"("Error code"=w321) -> ("Error description"=→"GetFilter":string)
                        n154 = call "TRUEorFALSE.vi"("bool number"=w316) -> ("String"=→"Is Filter ?":string)
                        n155 = local write "SetFilter"(w327) -> ()
                        n156 = local write "SetFilterInfo"(w327) -> ()
                      }
                    }
                  }
                }
              }
              frame #9 {
                n157 = Or(x=w328, y="Set Accessory") -> (x .or. y?=w330:bool)
                n158 = case shown="True" w330 {
                  tunnel: w331 -> [_ w334]
                  tunnel: "Set Accessory" -> [_ w333]
                  frame #0 {
                    n159 = Wait (ms)(milliseconds to wait=i32 ?) -> ()  [unwired: 1 out]
                  }
                  frame #1 {
                    n160 = stacked-sequence {
                      tunnel: w334 -> [w337 w347]
                      tunnel: w333 -> [w340 _]
                      frame #0 {
                        n161 = call "shamrock_accessoryAction.vi"("State"="State", "Line"="Line", "Set Accessory"=w340, "Device No"=w337) -> ("SetAccessory"=w336:u32)
                        n162 = call "code translator.vi"("Error code"=w336) -> ("Error description"=→"SetAccessory":string)
                      }
                      frame #1 {
                        n163 = call "shamrock_accessory.vi"("Device No"=w347) -> ("Line 2"=→"Line 2":i32, "Line 1"=→"Line 1":i32, "Line 1 & Line 2"=w344:u32, "0:FALSE / 1:TRUE"=w342:i32, "AccessoryIsPresent"=w345:u32)
                        n164 = call "code translator.vi"("Error code"=w345) -> ("Error description"=→"AccessoryIsPresent":string)
                        n165 = call "code translator.vi"("Error code"=w344) -> ("Error description"=→"GetAccessory":string)
                        n166 = call "TRUEorFALSE.vi"("bool number"=w342) -> ("String"=→"Is Accessory ?":string)
                        n167 = local write "Set Accessory"(bool ?) -> ()
                      }
                    }
                  }
                }
              }
              frame #10 {
                n168 = case shown="True" "Set Params" {
                  tunnel: w355 -> [_ w360]
                  tunnel: "Focal tilt" -> [_ w359]
                  tunnel: "Angular deviation" -> [_ w358]
                  tunnel: "Focal length" -> [_ w357]
                  frame #0 {
                    n169 = local write "Initializing"(bool ?) -> ()
                  }
                  frame #1 {
                    n170 = stacked-sequence {
                      tunnel: w360 -> [_ w367]
                      tunnel: w359 -> [_ w364]
                      tunnel: w358 -> [_ w363]
                      tunnel: w357 -> [_ w362]
                      frame #0 {
                        n171 = local write "Initializing"(bool ?) -> ()
                      }
                      frame #1 {
                        n172 = call "shamrock_setopticalparams.vi"("Focal Tilt"=w364, "Angular Deviation"=w363, "Focal Length"=w362, "Device No"=w367) -> ("SetOpticalParameters"=w366:u32)  [unwired: 7 in]
                        n173 = call "code translator.vi"("Error code"=w366) -> ("Error description"=→"Set Optical Parameters":string)
                      }
                    }
                  }
                }
              }
            }
          }
        }
      }
    }
    frame #3 {
      n174 = call "shamrock_close.vi"() -> ("Close"=w369:u32)
      n175 = call "code translator.vi"("Error code"=w369) -> ("Error description"=→"Close":string)
    }
  }
